vi "GetAcceleration.vi"(8 "error in (no error)":errorcluster, 11 "VISA resource name":refnum<visa-resource-name>) -> (0 "error out":errorcluster, 2 "Acceleration":dbl[](array[numeric]))   [LabVIEW 2014, in "GRBLMotionCore.lvlib"]
doc: "Performs an instrument error query before terminating the software connection to the instrument."
uses:
  <instrlib>/GRBL/GRBLMotionCore.lvlib
  <vilib>/Utility/error.llb/DialogType.ctl
  <vilib>/regexp/Match Regular Expression.xnode
panel:
  out "Read Buffer":string
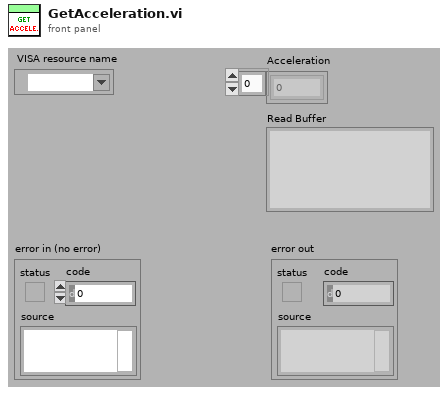
[diagram p1: front panel]
types:
  T1 = typedef "DialogType.ctl" = u16
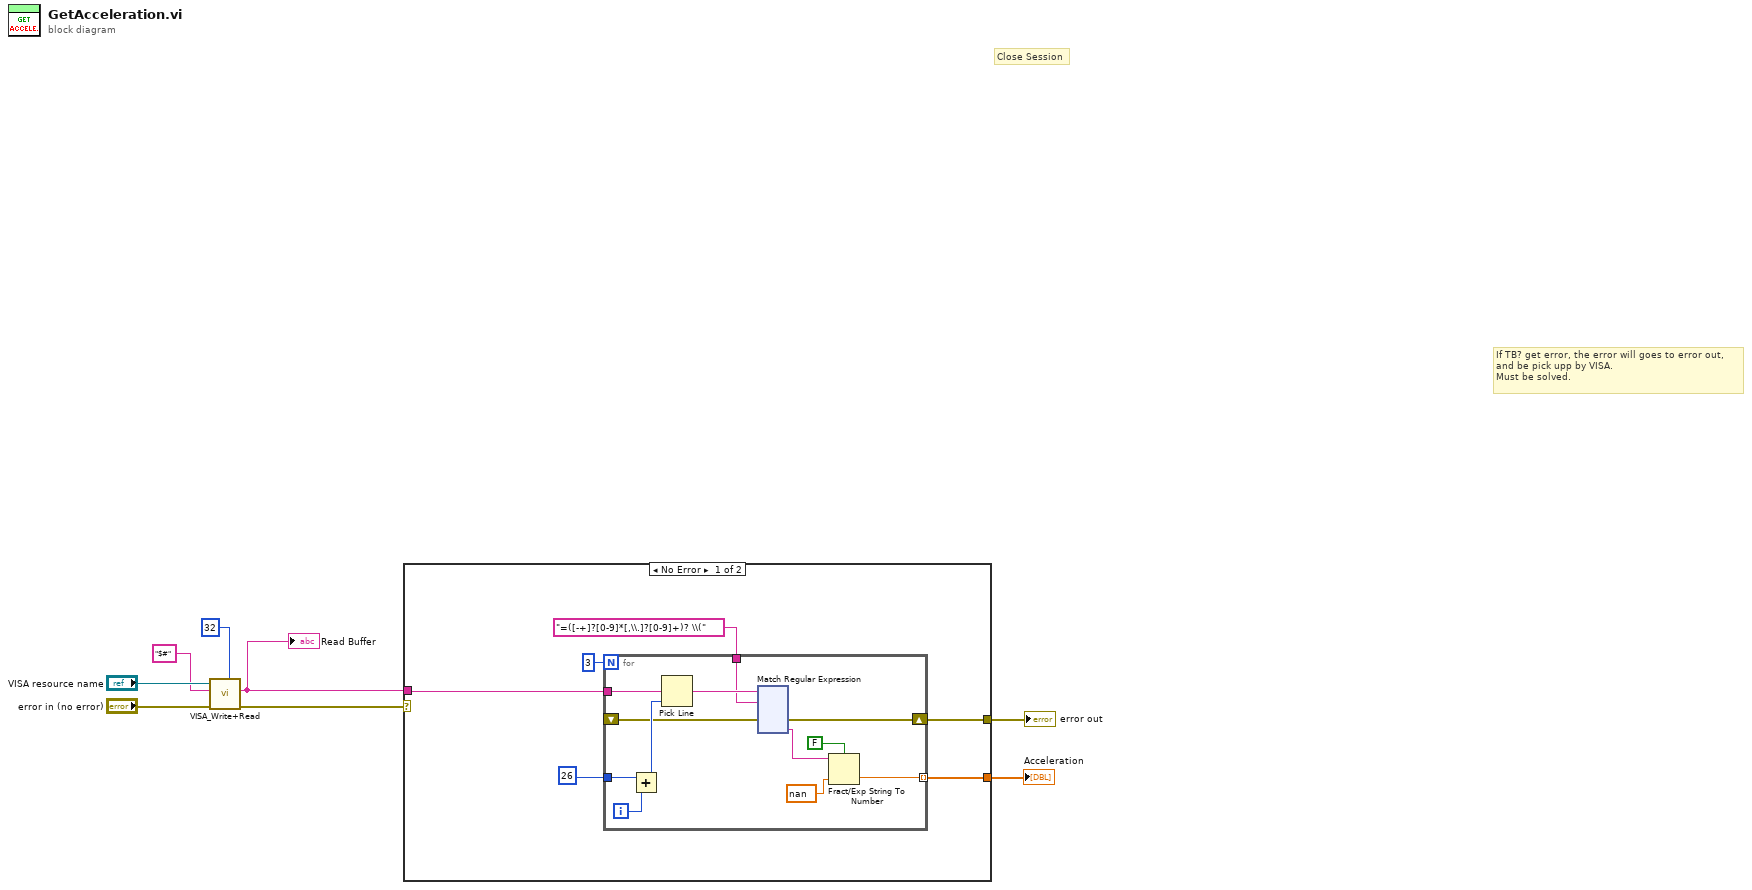
[diagram p0: block diagram]
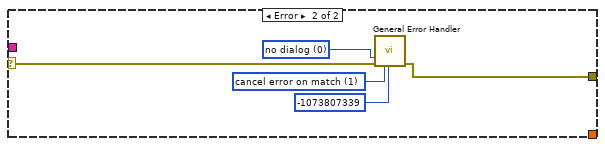
[diagram p2: hidden frame]
diagram:
  # "If TB? get error, the error will goes to error out, \nand be pick upp by VISA.\nMust be solved."
  # "Close Session"
  n1 = call <instrlib>:"VISA_Write+Read.vi"("NumRead"=32, "error in (no error)"="error in (no error)", "Write Buffer"="$#" ("string"), "VISA resource name"="VISA resource name") -> ("error out"=w4:errorcluster, "readout"=w5:string)  [unwired: 5 in, 1 out]
  "Read Buffer" <- w5
  n2 = case shown="No Error" w4 {
    selector: w4 -> [_ w142]
    tunnel: w5 -> [w11 _]
    tunnel: [w14 w143] -> w6
    tunnel: [w13 _] -> w1
    frame No Error {
      n3 = for {
        N: 3 -> [_]
        tunnel: [w22] -> w13 mode=indexing
        tunnel: w11 -> [w21]
        tunnel: 26 ("line index") -> [w18]
        tunnel: "=([-+]?[0-9]*[,\\.]?[0-9]+)? \\(" ("regular expression") -> [w16]
        shift-right: [w23] -> w14
        shift-left: _ -> [w15]
        i -> [w19]
        n4 = Add(x=w18, y=w19) -> (x+y=w17:i32)
        n5 = Pick Line(multi-line string=w21, line index=w17) -> (output string=w20:string)  [unwired: 1 in]
        n6 = xnode "Match Regular Expression"("input string"=w20, "regular expression"=w16, "error in"=w15) -> ("error out"=w23:errorcluster, "submatch 1"=w26:string)  [unwired: 3 in, 4 out]
        n7 = Fract/Exp String To Number(use system decimal point (T)=FALSE, string=w26, default (0 dbl)=nan ("default value 1")) -> (number=w22:dbl)  [unwired: 1 in, 1 out]
      }
    }
    frame Error {
      w140 = T1 0 items=["no dialog", "OK message", "continue or stop message", "OK message + warnings", "continue/stop + warnings"] ("type of dialog (OK msg:1)")
      w144 = 1 items=["no exception", "cancel error on match", "set error on match"] ("[exception action] (none:0)")
      n8 = call <vilib>:"General Error Handler.vi"("type of dialog (OK msg:1)"=w140, "error in (no error)"=w142, "[exception action] (none:0)"=w144, "[exception code]"=-1073807339) -> ("error out"=w143:errorcluster)  [unwired: 7 in, 4 out]
    }
  }
  "error out" <- w6
  "Acceleration" <- w1
